vi "LightSwitch (SubVI).vi"(4 "Stave Gain":dbl=16.0, 6 "Si Gain":dbl=2.0, 7 "Power Supply GPIB Address":string="8", 8 "error in":errorcluster, 10 "Spotlight":bool, 11 "Primary light":bool=TRUE) -> (0 "error out":errorcluster, 3 "Assigned camera gain":dbl)   [LabVIEW 2016]
doc: "Send commands with the GPIB Write function. Read the response from the instrument with the GPIB Read function.\n\nThis VI turns the lights on and off, and as such, it only sends voltage-related commands. We cannot independently turn off the lights using the \"output\" commands, since that cuts power for all channels. Thus, the \"OFF\" state will correspond to 0V supplied on the related channel. \n\nThe power supply is compatible with IEEE-488/2 and SCPI standards according to the manufacturer. Commands take the form of writes or queries. Semicolon, ';', concatenates commands.\n\n\nOverview: Turns the lights connected to the camera mount on and off. Built from the \"Simple GPIB\" NI example. (Demonstrates the use of the GPIB functions to communicate to a GPIB instrument.)\n\nRequirements: NI-488.2 Driver\nInstructions:\nEnsure the programmable power supply (GW Instek's PST-3202) is connected with the specified GPIB Address matching the control. Configure properly through Measurement & Automation Explorer.\n\nIn this VI, we assume that the primary light source is connected to the power supply via Channel 1, while the secondary light source, the spotlight, is connected on Channel 2. Our commands translate as follows: \n\nCHAN1:VOLT 7.0; VOLT? -- Set the voltage on channel 1 to 7.0 V, then check the voltage setting. We are not measuring the true voltage with this set up -- only the setting. Another VI, _______, serves as the slow control for monitoring the output voltage. An additional VI, ConfigureLights, configures the channels with the appropriate current, overcurrent and overvoltage protections."
panel:
  out "Response":string
  # "Overview: Turns the lights connected to the camera mount on and off.  Built from the \"Simple GPIB\" NI example. (Demonstrates the use of the GPIB functions to communicate to a GPIB instrument.)\n\nRequirements: NI-488.2 Driver\nInstructions:\nEnsure the programmable power supply (GW Instek's PST-3202) is connected with the specified GPIB Address matching the control. Configure properly through Measurement & Automation Explorer."
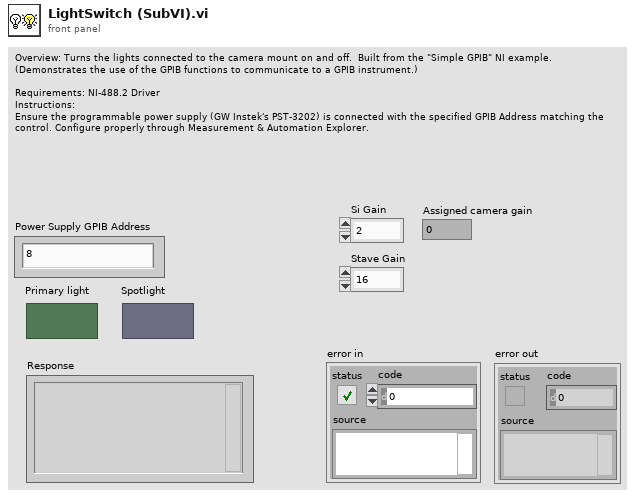
[diagram p1: front panel]
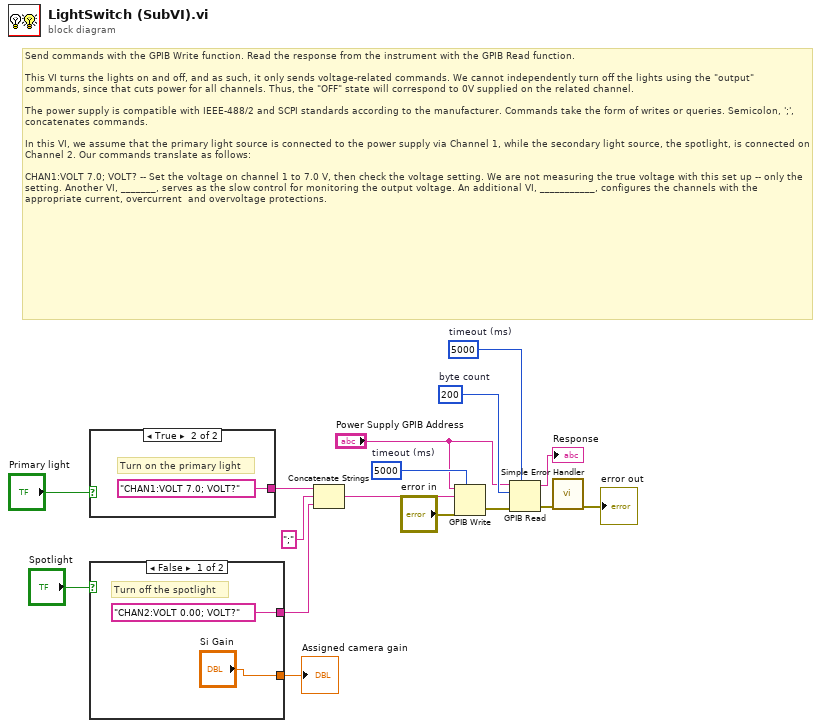
[diagram p0: block diagram]
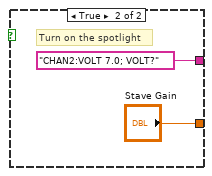
[diagram p2: hidden frame]
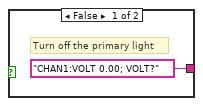
[diagram p3: hidden frame]
diagram:
  w10 = 5000  # timeout (ms)
  w13 = 200  # byte count
  w12 = 5000  # timeout (ms)
  # "Send commands with the GPIB Write function. Read the response from the instrument with the GPIB Read function.\n\nThis VI turns the lights on and off, and as such, it only sends voltage-related commands. We cannot independently turn off the lights using the \"output\" commands, since that cuts power for all channels. Thus, the \"OFF\" state will correspond to 0V supplied on the related channel. \n\nThe power supply is compatible with IEEE-488/2 and SCPI standards according to the manufacturer. Commands take the form of writes or queries. Semicolon, ';', concatenates commands.\n\nIn this VI, we assume that the primary light source is connected to the power supply via Channel 1, while the secondary light source, the spotlight, is connected on Channel 2. Our commands translate as follows: \n\nCHAN1:VOLT 7.0; VOLT? -- Set the voltage on channel 1 to 7.0 V, then check the voltage setting. We are not measuring the true voltage with this set up -- only the setting. Another VI, _______, serves as the slow control for monitoring the output voltage. An additional VI, ___________, configures the channels with the appropriate current, overcurrent  and overvoltage protections."
  n1 = case shown="True" "Primary light" {
    tunnel: ["CHAN1:VOLT 0.00; VOLT?" ("Characters to Write") "CHAN1:VOLT 7.0; VOLT?" ("Characters to Write")] -> w8
    frame False {
      # "Turn off the primary light"
    }
    frame True {
      # "Turn on the primary light"
    }
  }
  n2 = case shown="False" "Spotlight" {
    tunnel: ["CHAN2:VOLT 0.00; VOLT?" ("Characters to Write") "CHAN2:VOLT 7.0; VOLT?" ("Characters to Write")] -> w5
    tunnel: ["Si Gain" "Stave Gain"] -> w1
    frame False {
      # "Turn off the spotlight"
    }
    frame True {
      # "Turn on the spotlight"
    }
  }
  "Assigned camera gain" <- w1
  n3 = Concatenate Strings(w8, ";" ("string"), w5) -> (w4:string)
  n4 = GPIB Write(0:"Power Supply GPIB Address", 1:w4, 3:"error in", 4:w12) -> (6:w15:errorcluster)  [unwired: 1 in, 1 out]
  n5 = GPIB Read(0:"Power Supply GPIB Address", 1:w13, 3:w15, 4:w10) -> (5:→"Response":string, 7:w14:errorcluster)  [unwired: 1 in, 1 out]
  n6 = call <vilib>:"Simple Error Handler.vi"("error in (no error)"=w14) -> ("error out"=→"error out":errorcluster)  [unwired: 4 in, 4 out]
